vi "Fundamental Vector (1 Channel).vi"(8 "error in (no error)":errorcluster, 10 "current waveform":waveform(dbl), 11 "voltage waveform":waveform(dbl)) -> (0 "error out":errorcluster, 2 "current fundamental vector":cdb, 3 "voltage fundamental vector":cdb, 5 "frequency":dbl)   [LabVIEW 2014, in "NI_EP_Basic.lvlib"]
doc: "Calculates the fundamental vector of a voltage or current signal. Wire data to the <B>voltage waveform</B> input or the <B>current waveform</B> input to determine the polymorphic instance to use or manually select the instance."
uses:
  <vilib>/addons/Electrical Power/Basic/NI_EP_Basic.lvlib
  <vilib>/measure/matone.llb/Extract Single Tone Information 1 Chan.vi
  <vilib>/measure/NI_MAPro.lvlib
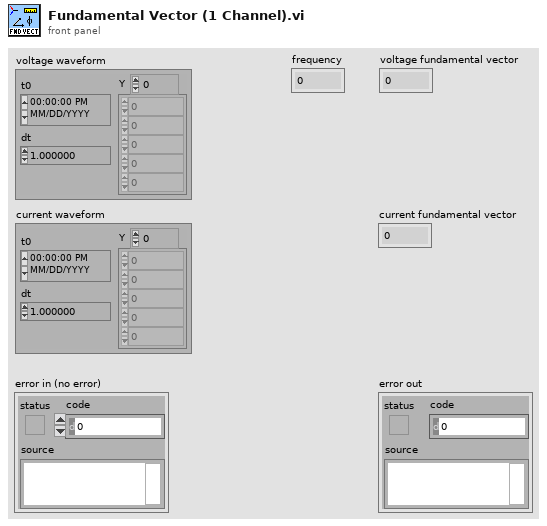
[diagram p1: front panel]
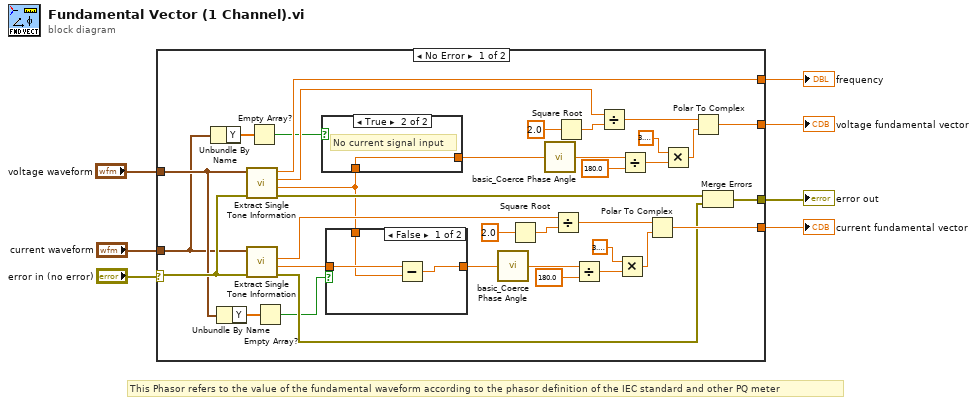
[diagram p0: block diagram]
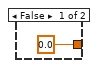
[diagram p2: hidden frame]
diagram:
  # "This Phasor refers to the value of the fundamental waveform according to the phasor definition of the IEC standard and other PQ meter"
  n1 = case shown="No Error" "error in (no error)" {
    selector: "error in (no error)" -> [w31 _]
    tunnel: "voltage waveform" -> [w15 _]
    tunnel: [w17 _] -> w2
    tunnel: [w33 _] -> w6
    tunnel: [w32 _] -> w3
    tunnel: "current waveform" -> [w11 _]
    tunnel: [w20 _] -> w4
    frame No Error {
      n2 = Unbundle By Name(w11) -> ("Y"=w12:dbl[])
      n3 = Unbundle By Name(w15) -> ("Y"=w14:dbl[])
      n4 = call-poly <vilib>:"Extract Single Tone Information.vi"("error in (no error)"=w31, "time signal in"=w15) -> ("error out"=w18:errorcluster, "detected phase (deg)"=w8:dbl, "detected amplitude"=w34:dbl, "detected frequency"=w32:dbl)  [unwired: 2 in, 4 out]
      n5 = call-poly <vilib>:"Extract Single Tone Information.vi"("error in (no error)"=w31, "time signal in"=w11) -> ("error out"=w19:errorcluster, "detected phase (deg)"=w22:dbl, "detected amplitude"=w16:dbl)  [unwired: 2 in, 5 out]
      n6 = Empty Array?(array=w12) -> (empty?=w10:bool)
      n7 = Empty Array?(array=w14) -> (empty?=w13:bool)
      n8 = case shown="True" w10 {
        tunnel: [0.0 ("detected phase (deg)") w44] -> w9
        tunnel: w8 -> [_ w44]
        frame False {
        }
        frame True {
          # "No current signal input"
        }
      }
      n9 = case shown="False" w13 {
        tunnel: w22 -> [w47 w48]
        tunnel: [w46 w48] -> w21
        tunnel: w8 -> [w45 _]
        frame False {
          n10 = Subtract(x=w47, y=w45) -> (x-y=w46:dbl)
        }
        frame True {
          # "No voltage signal input"
        }
      }
      n11 = call <vilib>:"basic_Coerce Phase Angle.vi"("Phase Angle"=w21) -> ("Phase Angle (-180 to 180)"=w23:dbl)  [unwired: 4 in]
      n12 = Square Root(x=2.0) -> (sqrt(x)=w29:dbl)
      n13 = call <vilib>:"basic_Coerce Phase Angle.vi"("Phase Angle"=w9) -> ("Phase Angle (-180 to 180)"=w42:dbl)  [unwired: 4 in]
      n14 = Divide(x=w16, y=w29) -> (x/y=w30:dbl)
      n15 = Square Root(x=2.0) -> (sqrt(x)=w36:dbl)
      n16 = Divide(x=w23, y=180.0) -> (x/y=w25:dbl)
      n17 = Divide(x=w34, y=w36) -> (x/y=w35:dbl)
      n18 = Multiply(x=3.141592653589793, y=w25) -> (x*y=w27:dbl)
      n19 = Divide(x=w42, y=180.0) -> (x/y=w40:dbl)
      n20 = Polar To Complex(1:w27, 2:w30) -> (0:w20:cdb)
      n21 = Multiply(x=3.141592653589793, y=w40) -> (x*y=w38:dbl)
      n22 = Polar To Complex(1:w38, 2:w35) -> (0:w33:cdb)
      n23 = Merge Errors(w18, w19) -> (w17:errorcluster)
    }
    frame Error {
    }
  }
  "voltage fundamental vector" <- w6
  "current fundamental vector" <- w4
  "error out" <- w2
  "frequency" <- w3
